vi "ConvertCompass.vi"(1 "Numeric":dbl) -> (0 "Heading from East":dbl)   [LabVIEW 2013]
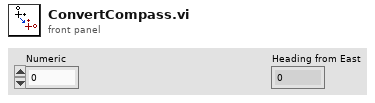
[diagram p1: front panel]
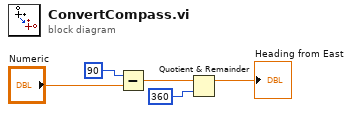
[diagram p0: block diagram]
diagram:
  n1 = Subtract(x=90, y="Numeric") -> (x-y=w3:dbl)
  n2 = Quotient & Remainder(x=w3, y=360) -> (x-y*floor(x/y)=→"Heading from East":dbl)  [unwired: 1 out]
